vi "nominal ingest tabular exclude column.vi"(8 "error in (no error)":errorcluster, 10 "column":string, 11 "staging":i32) -> (0 "error out":errorcluster, 3 "function return":i32)   [LabVIEW 2020, in "client.lvlib"]
doc: "int32_t nominal_ingest_tabular_exclude_column(int32_t staging, const char *column);"
uses:
  client.lvlib
  bin/nominalClient_64.dll
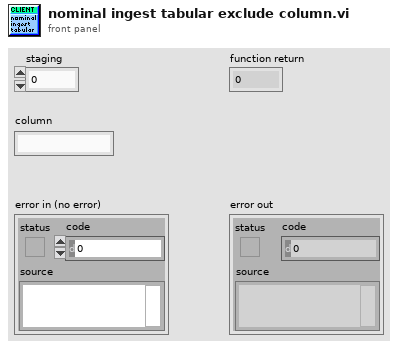
[diagram p1: front panel]
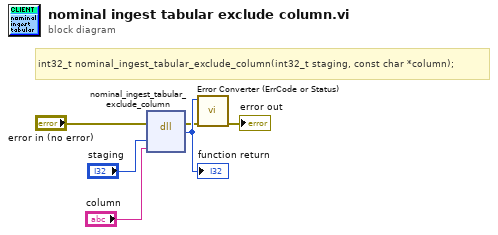
[diagram p0: block diagram]
diagram:
  # "int32_t nominal_ingest_tabular_exclude_column(int32_t staging, const char *column);"
  n1 = dll-call lib="C:/code/labview-client-rs/lv_src/bin/nominalClient_*.*" fn="nominal_ingest_tabular_exclude_column"(error in="error in (no error)", "staging"="staging", "column"="column") -> (error out=w2:errorcluster, w6:i32)  [unwired: 4 in, 1 out]
  "function return" <- w6
  n2 = call "Error Converter (ErrCode or Status).vi"("error in (no error)"=w2, "error code"=w6) -> ("error out"=→"error out":errorcluster)  [unwired: 9 in]
